vi "test.vi"() -> ()   [LabVIEW 2019]
panel:
  in  "stop":bool
  out "Image":T1(plugin-control)
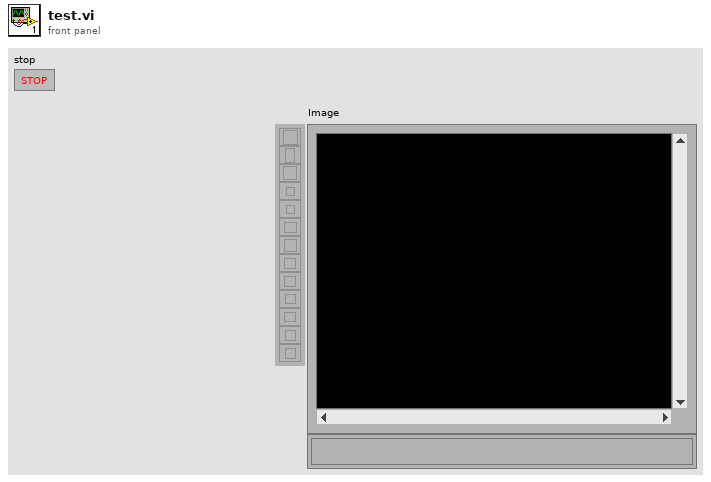
[diagram p1: front panel]
types:
  T1 = typedef "IMAQ Image.ctl" = refnum<image>
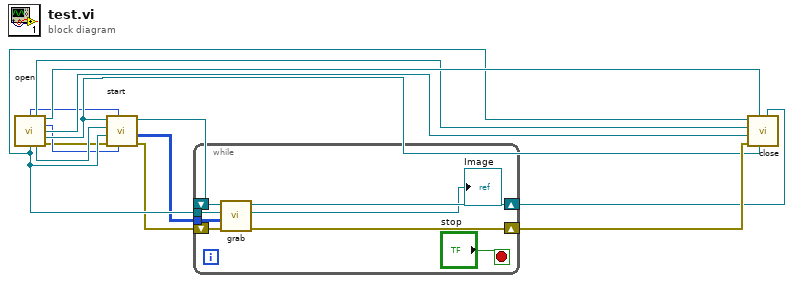
[diagram p0: block diagram]
diagram:
  n1 = call "open.vi"() -> ("w"=w2:i32, "SystemIdVarPtr"=w12:refnum<k24>, "ContextAppVarPtr"=w14:refnum<k24>, "h"=w5:i32, "DisplayIdVarPtr"=w7:refnum<k24>, "DigitizerIdVarPtr"=w6:refnum<k24>, "Mbuf"=w11:refnum<k24>, "new reference"=w10:refnum<k24>, "error out"=w4:errorcluster)  [unwired: 7 in]
  n2 = call "start.vi"("h"=w5, "w"=w2, "error in (no error)"=w4, "Mbuf"=w11, "new reference in"=w10, ".NET Refnum in"=w6) -> ("error out"=w3:errorcluster, "buf out"=w1:u16[][], ".NET Refnum out"=w9:refnum<k24>)  [unwired: 3 in]
  n3 = while {
    tunnel: w11 -> [w21]
    tunnel: w1 -> [w17]
    shift-right: [w19] -> w8
    shift-left: w9 -> [w20]
    shift-right: [w22] -> w13
    shift-left: w3 -> [w18]
    stop <- "stop" stop-if-true
    n4 = call "grab.vi"("error in (no error)"=w18, "buf in"=w17, "Mbuf"=w21, ".NET Refnum in"=w20) -> ("error out"=w22:errorcluster, "Image Out"=→"Image":T1, ".NET Refnum out"=w19:refnum<k24>)  [unwired: 5 in]
  }
  n5 = call "close.vi"(5:".NET Refnum in"=w8, "DigitizerIdVarPtr"=w6, "ContextAppVarPtr"=w14, "error in (no error)"=w13, "DisplayIdVarPtr"=w7, "SystemIdVarPtr"=w12, 11:".NET Refnum in"=w11) -> ()  [unwired: 4 in, 1 out]
